vi "OPC UA Client-Write - 2 Tags.vi"() -> ()   [LabVIEW 2017]
uses:
  <vilib>/OPCUA/controls/NodeId.ctl
  <vilib>/OPCUA/controls/Write Status.ctl
  <vilib>/OPCUA/client/Multiple Write Double.vi
  <vilib>/OPCUA/NI OPC UA Client.lvlib
panel:
  out "Temperature Fahrenheit":dbl=73.4
  in  "Node Id 2":string="Process Data.TemperatureF"
  in  "Node Id":string="Process Data.TemperatureC"
  in  "Stop Button":bool
  in  "Temperature Celsius":dbl=23.0
  in  "Server Endpoint URL":string="opc.tcp://XPS15HPH:49580"
  # "F"
  # "C"
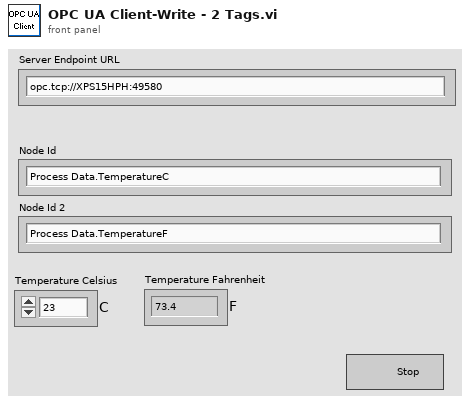
[diagram p1: front panel]
types:
  T1 = cluster{"message mode":enum16{"None", "Sign", "Sign and Encrypt"}, "security":enum16{"Basic256", "Basic128Rsa15"}}
  T2 = typedef "OPC UA Client Refnum.ctl" = refnum<k21>
  T3 = typedef "NodeId.ctl" = string
  T4 = typedef "Write Status.ctl" = u32
  T5 = cluster{"node ID":T3, "value":dbl, "timestamp (current time)":timestamp, "node status":T4}
  T6 = cluster{"node ID":T3, "value":dbl, "timestamp (current time)":timestamp, "node status":T4}[]
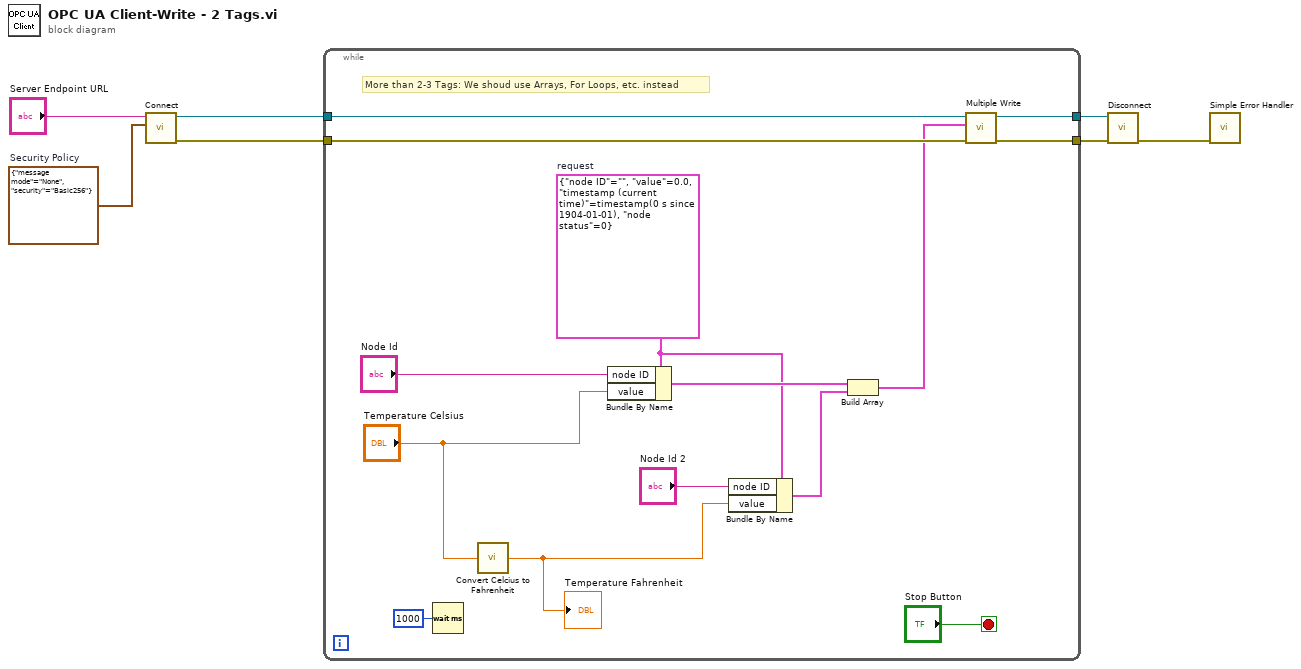
[diagram p0: block diagram]
diagram:
  w1 = T1 {"message mode"=enum."None", "security"=enum."Basic256"}  # Security Policy
  n1 = call <vilib>:"Connect.vi"("security policy"=w1, "server endpoint URL"="Server Endpoint URL") -> ("error out"=w6:errorcluster, "OPC UA client refnum out"=w7:T2)  [unwired: 7 in, 1 out]
  n2 = while {
    tunnel: w7 -> [w19]
    tunnel: w6 -> [w18]
    tunnel: [w17] -> w5
    tunnel: [w16] -> w3
    stop <- "Stop Button" stop-if-true
    w11 = T5 {"node ID"="", "value"=0.0, "timestamp (current time)"=timestamp(0 s since 1904-01-01), "node status"=0}  # request
    # "More than 2-3 Tags: We shoud use Arrays, For Loops, etc. instead"
    n3 = Wait (ms)(milliseconds to wait=u32 1000) -> ()  [unwired: 1 out]
    n4 = call "Convert Celcius to Fahrenheit.vi"("Tc"="Temperature Celsius") -> ("Tf"=w9:dbl)
    "Temperature Fahrenheit" <- w9
    n5 = Bundle By Name(cluster=w11, "node ID"="Node Id", "value"="Temperature Celsius") -> (w14:T5)
    n6 = Bundle By Name(cluster=w11, "node ID"="Node Id 2", "value"=w9) -> (w12:T5)
    n7 = Build Array "Build Array"(w14, w12) -> (w8:T6)
    n8 = call-poly <vilib>:"Multiple Write.vi"("error in (no error)"=w18, "requests"=w8, "OPC UA client refnum in"=w19) -> ("error out"=w16:errorcluster, "OPC UA client refnum out"=w17:T2)  [unwired: 5 in, 2 out]
  }
  n9 = call <vilib>:"Disconnect.vi"("error in (no error)"=w3, "OPC UA client refnum in"=w5) -> ("error out"=w4:errorcluster)  [unwired: 9 in]
  n10 = call <vilib>:"Simple Error Handler.vi"("error in (no error)"=w4) -> ()  [unwired: 4 in, 5 out]
